vi "find robot location.vi"(6 "Reverse?":bool, 8 "Pigeon Reference":T2={"DeviceStatus"={"status"=FALSE, "code"=0, "source"=""}, "Device Number"=0, "Type"=352321536, "Device ID"=0, "Handle"=0, "UsageFrame"=0, "Library Path"=path ""} {"Type" items=["CAN"=352321536, "TalonSRX"=33554432]}, 9 "Right Encoder Reference":T4={"DeviceStatus"={"status"=FALSE, "code"=0, "source"=""}, "Type"=enum."PWM", "PWM"={"PWM Channel"=enum."Invalid", "DeadBand"={"Name"="", "maxPositivePwm"=0, "minPositivePwm"=0, "centerPwm"=0, "maxNegativePwm"=0, "minNegativePwm"=0, "angularRange"=0}}, "CAN"={"Device Number"=0, "SetOutput VI Ref"=variant(enum8{"Percent VBus", "Current", "Speed", "Position", "Voltage"} enum."Percent VBus"), "GetOutput VI Ref"=variant(refnum<k1> refnum), "Enable VI Ref"=variant(dbl 12.0), "Disable VI Ref"=variant(enum8{"Percent VBus", "Speed", "Position", "Slave", "Unchanged / Invalid", "Voltage Compensation", "Current", "Motion Profile"} enum."Percent VBus"), "Data"=variant}, "Invert"=FALSE, "DIO PWM"={"PWM \"Enable\" Channel"=enum."Invalid", "DIOChannel"=enum."Invalid", "PWM Rate"=0.0}}, 10 "Left Encoder Reference":T4={"DeviceStatus"={"status"=FALSE, "code"=0, "source"=""}, "Type"=enum."PWM", "PWM"={"PWM Channel"=enum."Invalid", "DeadBand"={"Name"="", "maxPositivePwm"=0, "minPositivePwm"=0, "centerPwm"=0, "maxNegativePwm"=0, "minNegativePwm"=0, "angularRange"=0}}, "CAN"={"Device Number"=0, "SetOutput VI Ref"=variant(enum8{"Percent VBus", "Current", "Speed", "Position", "Voltage"} enum."Percent VBus"), "GetOutput VI Ref"=variant(refnum<k1> refnum), "Enable VI Ref"=variant(dbl 12.0), "Disable VI Ref"=variant(enum8{"Percent VBus", "Speed", "Position", "Slave", "Unchanged / Invalid", "Voltage Compensation", "Current", "Motion Profile"} enum."Percent VBus"), "Data"=variant}, "Invert"=FALSE, "DIO PWM"={"PWM \"Enable\" Channel"=enum."Invalid", "DIOChannel"=enum."Invalid", "PWM Rate"=0.0}}, 11 "Path Data":T1={"Path"=[], "Target Velocities"=[], "Robot Location"=[], "Relative Robot Angle (rad)"=0.0, "Curvature"=0.0, "Lookahead Point"=[3064.399009129367, 18229.833030071386], "Lookahead Index"=8.422809037111724, "Closest Point"=[], "Closest Point Index"=0, "Left Velocity"=0.0, "Right Velocity"=0.0, "Left Encoder Vel"=0, "Right Encoder Vel"=0, "Left Encoder Pos"=0, "Right Encoder Pos"=0, "Inital Robot Angle (deg)"=0.0}) -> (3 "Path Data":T1={"Path"=[], "Target Velocities"=[], "Robot Location"=[], "Relative Robot Angle (rad)"=0.0, "Curvature"=0.0, "Lookahead Point"=[3064.399009129367, 18229.833030071386], "Lookahead Index"=8.422809037111724, "Closest Point"=[], "Closest Point Index"=0, "Left Velocity"=0.0, "Right Velocity"=0.0, "Left Encoder Vel"=0, "Right Encoder Vel"=0, "Left Encoder Pos"=0, "Right Encoder Pos"=0, "Inital Robot Angle (deg)"=0.0})   [LabVIEW 2018]
uses:
  <vilib>/Rock Robotics/WPI/MotorControl/WPI_MotorControlDeviceRef.ctl
  <vilib>/Rock Robotics/WPI/MotorControl/WPI_MotorControlType.ctl
  <vilib>/Rock Robotics/SystemInterfaces/DIO/FPGA_DIOPWMChannel.ctl
  <vilib>/Rock Robotics/WPI/PWM/WPI_PWMDeadband.ctl
  <vilib>/Rock Robotics/SystemInterfaces/DIO/FPGA_DIOChannel.ctl
  <vilib>/Rock Robotics/WPI/ThirdParty/Phoenix-LabVIEW/Pigeon IMU/CTRE_PigeonIMU_DeviceRef.ctl
  <vilib>/Rock Robotics/WPI/ThirdParty/Phoenix-LabVIEW/Pigeon IMU/CTRE_PigeonIMU_ConnectionType.ctl
  path data.ctl
  <vilib>/Rock Robotics/WPI/ThirdParty/Phoenix-LabVIEW/Motor Controller/Get/CTRE_Phoenix_MotorController_GetQuadratureData.vi
  <vilib>/Rock Robotics/WPI/ThirdParty/Phoenix-LabVIEW/Pigeon IMU/CTRE_PigeonIMU_GetYPR.vi
panel:
  out "Robot Angle (rad)":dbl
  out "Robot Location":dbl[](array[numeric])
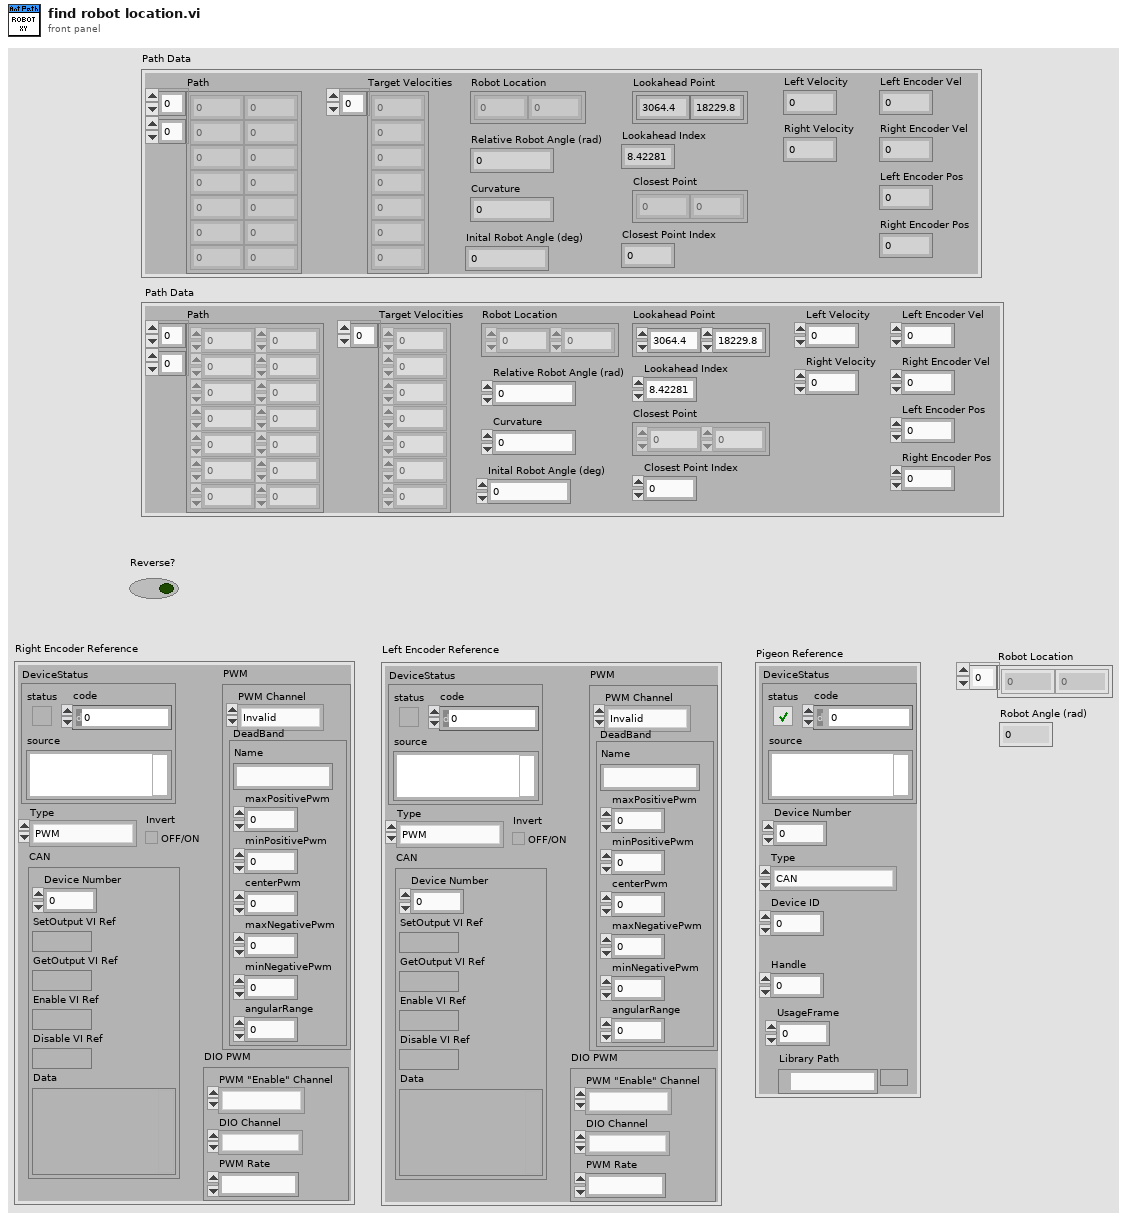
[diagram p1: front panel]
types:
  T1 = typedef "path data.ctl" = cluster{"Path":dbl[][], "Target Velocities":dbl[], "Robot Location":dbl[], "Relative Robot Angle (rad)":dbl, "Curvature":dbl, "Lookahead Point":dbl[], "Lookahead Index":dbl, "Closest Point":dbl[], "Closest Point Index":i32, "Left Velocity":dbl, "Right Velocity":dbl, "Left Encoder Vel":i32, "Right Encoder Vel":i32, "Left Encoder Pos":i32, "Right Encoder Pos":i32, "Inital Robot Angle (deg)":dbl}
  T2 = typedef "CTRE_PigeonIMU_DeviceRef.ctl" = cluster{"DeviceStatus":errorcluster, "Device Number":u8, "Type":T3, "Device ID":u32, "Handle":u64, "UsageFrame":u32, "Library Path":path}
  T3 = typedef "CTRE_PigeonIMU_ConnectionType.ctl" = u32
  T4 = typedef "WPI_MotorControlDeviceRef.ctl" = cluster{"DeviceStatus":errorcluster, "Type":T5, "PWM":cluster{"PWM Channel":T6, "DeadBand":T7}, "CAN":cluster{"Device Number":u8, "SetOutput VI Ref":variant, "GetOutput VI Ref":variant, "Enable VI Ref":variant, "Disable VI Ref":variant, "Data":variant}, "Invert":bool, "DIO PWM":cluster{"PWM \"Enable\" Channel":T6, "DIOChannel":T8, "PWM Rate":dbl}}
  T5 = typedef "WPI_MotorControlType.ctl" = enum16{"PWM", "CAN", "DIO PWM"}
  T6 = typedef "FPGA_DIOPWMChannel.ctl" = enum8{"PWM 0", "PWM 1", "PWM 2", "PWM 3", "PWM 4", "PWM 5", "PWM 6", "PWM 7", "PWM 8", "PWM 9", "PWM MXP 0", "PWM MXP 1", "PWM MXP 2", "PWM MXP 3", "PWM MXP 4", "PWM MXP 5", "PWM MXP 6", "PWM MXP 7", "PWM MXP 8", "PWM MXP 9", "Invalid"}
  T7 = typedef "WPI_PWMDeadband.ctl" = cluster{"Name":string, "maxPositivePwm":i32, "minPositivePwm":i32, "centerPwm":i32, "maxNegativePwm":i32, "minNegativePwm":i32, "angularRange":u16}
  T8 = typedef "FPGA_DIOChannel.ctl" = enum8{"DIO 0", "DIO 1", "DIO 2", "DIO 3", "DIO 4", "DIO 5", "DIO 6", "DIO 7", "DIO 8", "DIO 9", "DIO MXP 0", "DIO MXP 1", "DIO MXP 2", "DIO MXP 3", "DIO MXP 4", "DIO MXP 5", "DIO MXP 6", "DIO MXP 7", "DIO MXP 8", "DIO MXP 9", "DIO MXP 10", "DIO MXP 11", "DIO MXP 12", "DIO MXP 13", "DIO MXP 14", "DIO MXP 15", "SPI Port CS1", "SPI Port CS2", "SPI Port CS3", "SPI Port MISO", "SPI Port MOSI", "Invalid"}
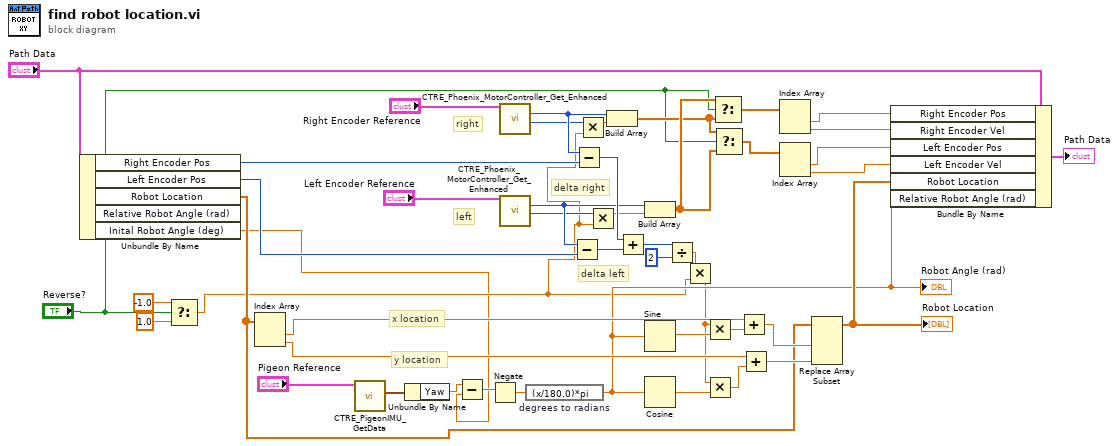
[diagram p0: block diagram]
diagram:
  # "left"
  # "right"
  # "delta left"
  # "delta right"
  # "x location"
  # "y location"
  n1 = Unbundle By Name("Path Data") -> ("Right Encoder Pos"=w27:i32, "Left Encoder Pos"=w26:i32, "Robot Location"=w25:dbl[], "Inital Robot Angle (deg)"=w1:dbl)  [unwired: 1 out]
  n2 = Select(t=-1.0, s="Reverse?", f=1.0) -> (s? t:f=w4:dbl)
  n3 = Index Array(array=w25) -> (element #1=w38:dbl, element #2=w37:dbl)  [unwired: 2 in]
  n4 = call-poly <vilib>:"CTRE_PigeonIMU_GetData.vi"("PigeonIMUDevRef"="Pigeon Reference") -> ("Yaw Pitch Roll"=w41:cluster{"Yaw":dbl, "Pitch":dbl, "Roll":dbl})  [unwired: 8 in, 2 out]
  n5 = Unbundle By Name(w41) -> ("Yaw"=w2:dbl)
  n6 = Subtract(x=w2, y=w1) -> (x-y=w3:dbl)
  n7 = Negate(x=w3) -> (-x=w40:dbl)
  n8 = call-poly <vilib>:"CTRE_Phoenix_MotorController_Get_Enhanced.vi"("PhoenixMotorControlDevRef"="Right Encoder Reference") -> ("Quadrature Position"=w19:i32, "Quadrature Velocity"=w18:i32)  [unwired: 11 in, 2 out]
  n9 = call-poly <vilib>:"CTRE_Phoenix_MotorController_Get_Enhanced.vi"("PhoenixMotorControlDevRef"="Left Encoder Reference") -> ("Quadrature Position"=w17:i32, "Quadrature Velocity"=w16:i32)  [unwired: 11 in, 2 out]
  n10 = expression code="(x/180.0)*pi" "degrees to radians"(w40) -> (w23:dbl)
  "Robot Angle (rad)" <- w23
  n11 = Subtract(x=w17, y=w26) -> (x-y=w33:i32)
  n12 = Subtract(x=w19, y=w27) -> (x-y=w34:i32)
  n13 = Multiply(x=w18, y=w4) -> (x*y=w5:dbl)
  n14 = Multiply(x=w16, y=w4) -> (x*y=w6:dbl)
  n15 = Build Array(w19, w5) -> (w14:dbl[])
  n16 = Add(x=w34, y=w33) -> (x+y=w32:i32)
  n17 = Build Array(w17, w6) -> (w15:dbl[])
  n18 = Sine(x=w23) -> (sin(x)=w45:dbl)
  n19 = Cosine(x=w23) -> (cos(x)=w44:dbl)
  n20 = Divide(x=w32, y=2) -> (x/y=w28:dbl)
  n21 = Multiply(x=w28, y=w4) -> (x*y=w20:dbl)
  n22 = Multiply(x=w20, y=w45) -> (x*y=w42:dbl)
  n23 = Multiply(x=w20, y=w44) -> (x*y=w43:dbl)
  n24 = Select(t=w15, s="Reverse?", f=w14) -> (s? t:f=w12:dbl[])
  n25 = Select(t=w14, s="Reverse?", f=w15) -> (s? t:f=w9:dbl[])
  n26 = Add(x=w38, y=w42) -> (x+y=w36:dbl)
  n27 = Add(x=w37, y=w43) -> (x+y=w35:dbl)
  n28 = Index Array(array=w12) -> (element #1=w11:dbl, element #2=w10:dbl)  [unwired: 2 in]
  n29 = Index Array(array=w9) -> (element #1=w8:dbl, element #2=w7:dbl)  [unwired: 2 in]
  n30 = Replace Array Subset(array=w25, new element #1=w36, new element #2=w35) -> (w24:dbl[])  [unwired: 2 in]
  "Robot Location" <- w24
  n31 = Bundle By Name(cluster="Path Data", "Right Encoder Pos"=w11, "Right Encoder Vel"=w10, "Left Encoder Pos"=w8, "Left Encoder Vel"=w7, "Robot Location"=w24, "Relative Robot Angle (rad)"=w23) -> (→"Path Data":T1)
